vi "Initialize Device Core.vi"(8 "error in (no error)":errorcluster, 9 "Reset (F)":bool, 10 "Resource Name":string, 11 "CS++DMM in":refnum<class "CS++DMM.lvclass">) -> (0 "error out":errorcluster, 3 "CS++DMM out":refnum<class "CS++DMM.lvclass">)   [LabVIEW 2013, in "CS++DMM.lvlib" / "CS++DMM.lvclass"]
doc: "Initialize device driver."
uses:
  CS++DMM.lvclass
  Core/Actors/CS++DeviceActor/CS++DeviceActor.lvclass
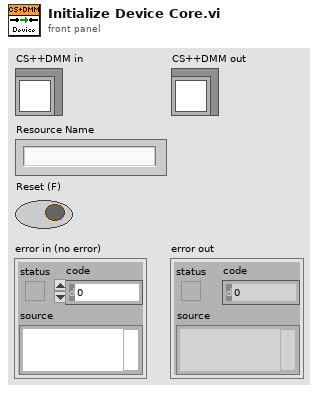
[diagram p1: front panel]
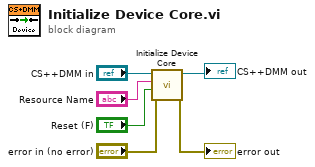
[diagram p0: block diagram]
diagram:
  n1 = call-parent "Initialize Device Core.vi"("error in (no error)"="error in (no error)", "Reset (F)"="Reset (F)", "Resource Name"="Resource Name", "CS++DeviceActor in"="CS++DMM in") -> ("error out"=→"error out":errorcluster, "CS++DeviceActor out"=→"CS++DMM out":refnum<class "CS++DMM.lvclass">)  [unwired: 6 in]
